vi "Delete Data.vi"(0 "VISA Resource Name":refnum<visa-resource-name>, 5 "File Type (2:SPECIFIED FILE)":T1(ring)=enum."SPECIFIED FILE", 9 "File Name (User_File)":string="USER_FILE", 11 "error in (no error)":errorcluster {"code" format="%.0x"}) -> (4 "VISA Resource Name Out":refnum<visa-resource-name>, 15 "error out":errorcluster {"code" format="%.0x"})   [LabVIEW 2012, in "Agilent ESG Series.lvlib"]
doc: "This VI is used delete files from the instrument memory."
uses:
  <instrlib>/Agilent ESG Series/Agilent ESG Series.lvlib
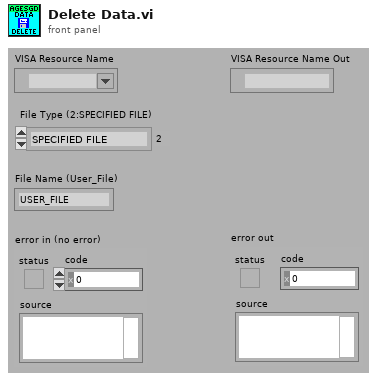
[diagram p1: front panel]
types:
  T1 = enum16{"ALL", "BINARY", "SPECIFIED FILE", "LIST", "STATE"}
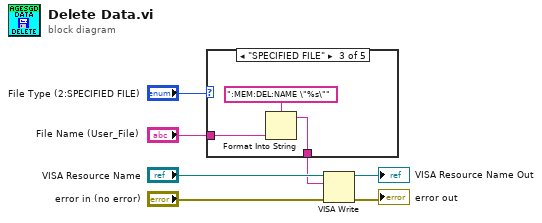
[diagram p0: block diagram]
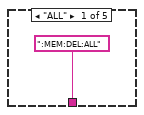
[diagram p2: hidden frame]
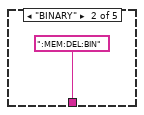
[diagram p3: hidden frame]
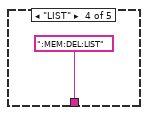
[diagram p4: hidden frame]
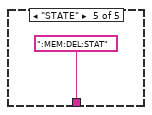
[diagram p5: hidden frame]
diagram:
  n1 = case shown="\"SPECIFIED FILE\"" "File Type (2:SPECIFIED FILE)" {
    tunnel: [":MEM:DEL:ALL" ":MEM:DEL:BIN" w11 ":MEM:DEL:LIST" ":MEM:DEL:STAT"] -> w5
    tunnel: "File Name (User_File)" -> [_ _ w10 _ _]
    frame "ALL" {
    }
    frame "BINARY" {
    }
    frame "SPECIFIED FILE" {
      n2 = Format Into String(format string=":MEM:DEL:NAME \"%s\"", w10) -> (resulting string=w11:string)  [unwired: 2 in, 1 out]
    }
    frame "LIST" {
    }
    frame "STATE" {
    }
  }
  n3 = VISA Write(VISA resource name="VISA Resource Name", write buffer=w5, error in (no error)="error in (no error)") -> (VISA resource name out=→"VISA Resource Name Out":refnum<visa-resource-name>, error out=→"error out":errorcluster)  [unwired: 1 out]
